vi "WhichVIsShouldRegenerate.vi"(8 "DoAllOfThem":bool, 10 "CommandTemplatesFolder":path=path "C:/Users/competition/Documents/LabVIEW Data/Projects/xml-auto-routine/CreateCommands/CommandTemplates", 11 "LastModifiedDatesFolder":path=path "C:/Users/competition/Documents/LabVIEW Data/Projects/xml-auto-routine/CreateCommands") -> (0 "New VI":bool, 2 "iniRefecence":T1, 3 "VINames":string[](array[string]))   [LabVIEW 2017]
uses:
  <vilib>/Utility/config.llb/Config Data RefNum.ctl
  <vilib>/Utility/config.llb/Read Key (String).vi
  <vilib>/Utility/config.llb/NI_LVConfig.lvlib
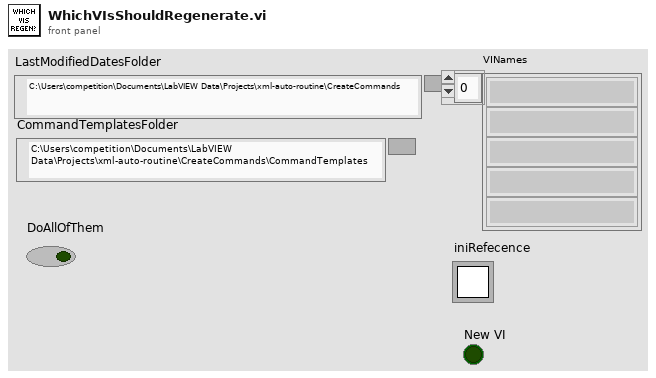
[diagram p1: front panel]
types:
  T1 = typedef "NI_LVConfig.lvlib/Config Data RefNum.ctl" = refnum<k1>
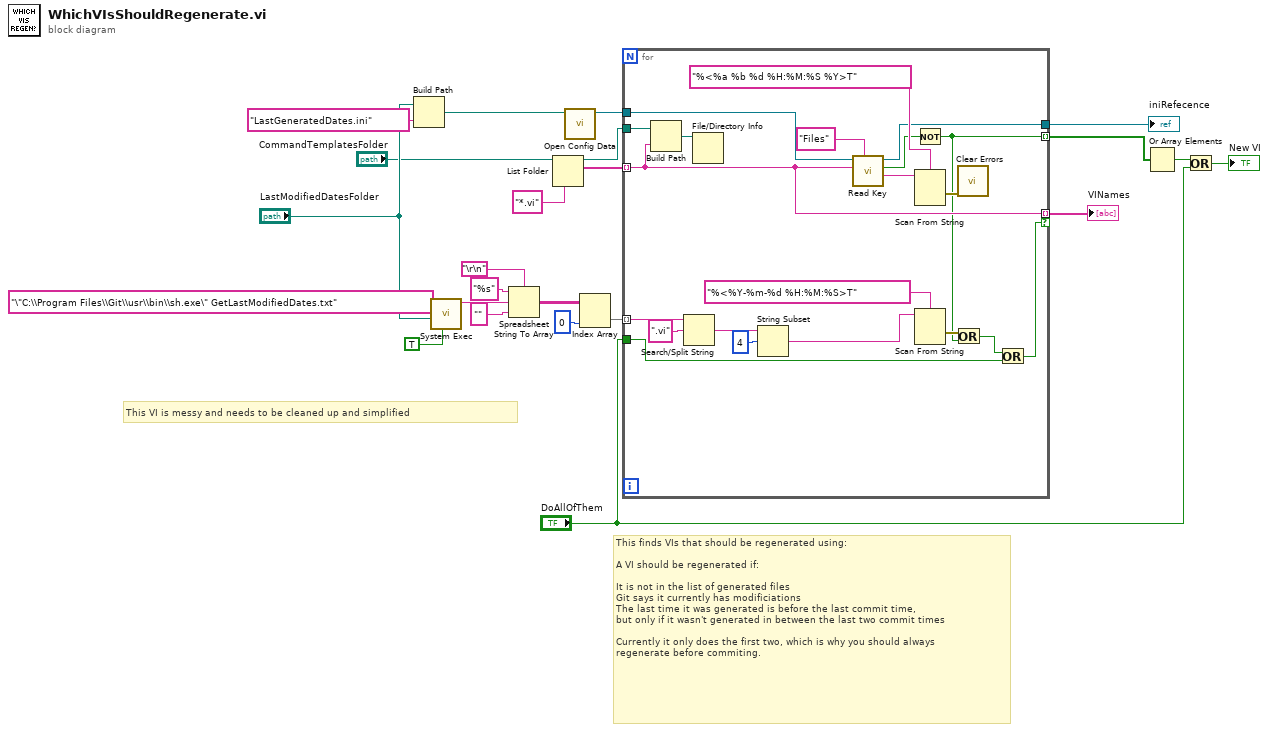
[diagram p0: block diagram]
diagram:
  # "This VI is messy and needs to be cleaned up and simplified"
  # "This finds VIs that should be regenerated using:\n\nA VI should be regenerated if:\n\nIt is not in the list of generated files\nGit says it currently has modificiations\nThe last time it was generated is before the last commit time,\nbut only if it wasn't generated in between the last two commit times\n\nCurrently it only does the first two, which is why you should always\nregenerate before commiting."
  n1 = Build Path(base path="LastModifiedDatesFolder", name or relative path="LastGeneratedDates.ini") -> (appended path=w17:path)
  n2 = call <vilib>:"System Exec.vi"("run minimized? (F)"=TRUE, "working directory"="LastModifiedDatesFolder", "command line"="\"C:\\Program Files\\Git\\usr\\bin\\sh.exe\" GetLastModifiedDates.txt") -> ("standard output"=w10:string)  [unwired: 5 in, 3 out]
  n3 = Spreadsheet String To Array(delimiter (Tab)="\r\n", format string="%s", spreadsheet string=w10, array type (2D Dbl)="" ("format string")) -> (array=w7:string[][])
  n4 = List Folder(path="CommandTemplatesFolder", pattern="*.vi") -> (path out=w14:path, filenames=w15:string[])  [unwired: 2 in, 2 out]
  n5 = call <vilib>:"Open Config Data.vi"("configuration file path"=w17) -> ("refnum"=w13:T1)  [unwired: 8 in, 2 out]
  n6 = Index Array(array=w7, index (col)=0 ("disabled index (col)")) -> (element=w5:string[])  [unwired: 1 in]
  n7 = for {
    tunnel: w15 -> [w38] mode=indexing
    tunnel: w14 -> [w40]
    tunnel: w13 -> [w39]
    tunnel: [w38] -> w12 mode=indexing if=w25
    tunnel: [w37] -> w11
    tunnel: w5 -> [w29] mode=indexing
    tunnel: "DoAllOfThem" -> [w26]
    tunnel: [w24] -> w4 mode=indexing
    n8 = Build Path(base path=w40, name or relative path=w38) -> (appended path=w41:path)
    n9 = Search/Split String(string=w29, search string/char (-)=".vi") -> (match + rest of string=w35:string)  [unwired: 1 in, 2 out]
    n10 = File/Directory Info(path=w41) -> ()  [unwired: 1 in, 7 out]
    n11 = String Subset(string=w35, offset (0)=4) -> (substring=w34:string)  [unwired: 1 in]
    n12 = call-poly <vilib>:"Read Key.vi"("section"="Files", "key"=w38, "refnum"=w39) -> ("value"=w44:string, "found?"=w31:bool, "refnum out"=w37:T1)  [unwired: 5 in, 1 out]
    n13 = Not(x=w31) -> (.not. x?=w24:bool)
    n14 = Scan From String(format string="%<%a %b %d %H:%M:%S %Y>T", input string=w44) -> (error out=w32:errorcluster)  [unwired: 4 in, 2 out]
    n15 = Scan From String(format string="%<%Y-%m-%d %H:%M:%S>T", input string=w34) -> (error out=w30:errorcluster)  [unwired: 4 in, 2 out]
    n16 = Or(x=w30, y=w24) -> (x .or. y?=w27:bool)
    n17 = call <vilib>:"Clear Errors.vi"("error in (no error)"=w32) -> ()  [unwired: 5 in, 2 out]
    n18 = Or(x=w27, y=w26) -> (x .or. y?=w25:bool)
  }
  "VINames" <- w12
  "iniRefecence" <- w11
  n19 = Or Array Elements(Boolean array=w4) -> (logical OR=w3:bool)
  n20 = Or(x=w3, y="DoAllOfThem") -> (x .or. y?=→"New VI":bool)
